vi "AuMT8852B Single Payload Frequency.vi"(5 "Frequency (2441 MHz)":dbl=2441.0, 7 "Set/Get (Set)":enum16{"Set", "Get"}(ring), 8 "error in (no error)":errorcluster, 9 "Type (TX)":enum16{"TX", "RX"}(ring), 10 "Script (3)":i32=3, 11 "VISA session":refnum<visa-resource-name>) -> (0 "error out":errorcluster, 2 "error code":i32, 3 "VISA session out":refnum<visa-resource-name>, 4 "Frequency out":dbl=2441.0)   [LabVIEW 2017]
doc: "Anritsu MT8850 Bluetooth Tester\n\nDetermines the TX or RX frequency for Bluetooth tests (Carrier, Sensitivity, etc.) whose scripts are set to Single Payload mode.\n\nINPUTS\n Set/Get - whether the value is being sent to or retrieved from the instrument.\n Script - the script to access.\n Type - whether the specified frequency is the TX or RX frequency.\n Frequency - value to be used in Single Payload mode.\n\nOUTPUTS\n Frequency out - value currently being used in Single Payload mode."
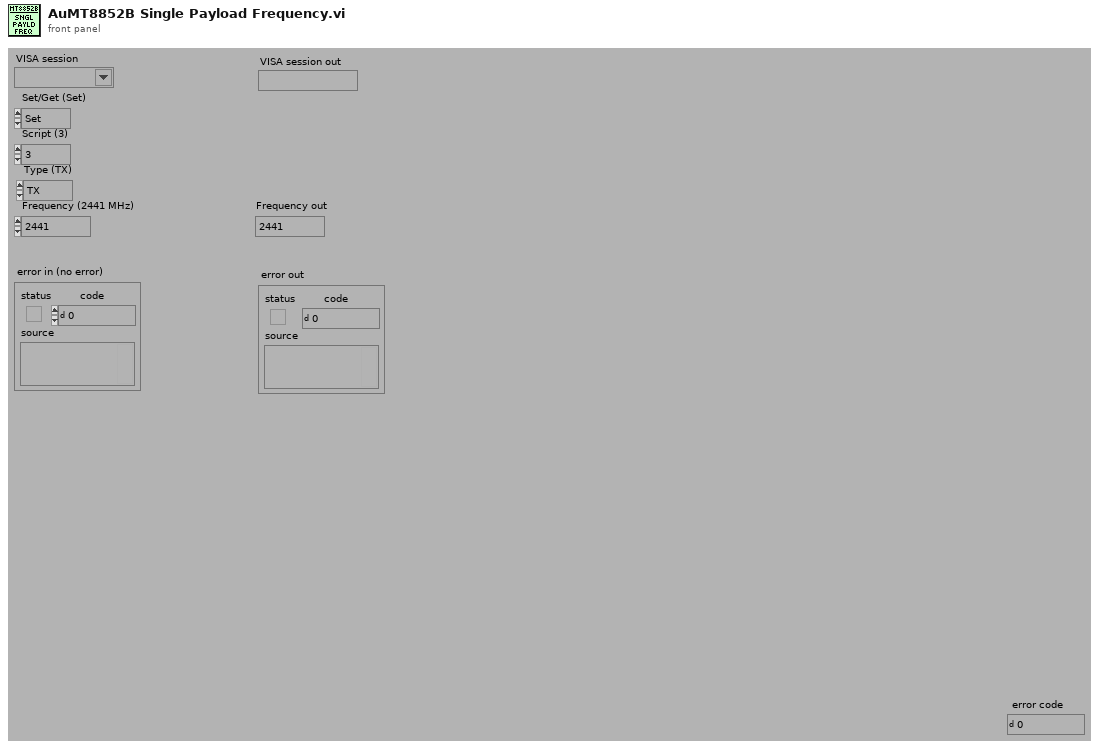
[diagram p1: front panel]
types:
  T1 = enum16{"Simulate", "Range check", "Cache", "Query instrument status"}
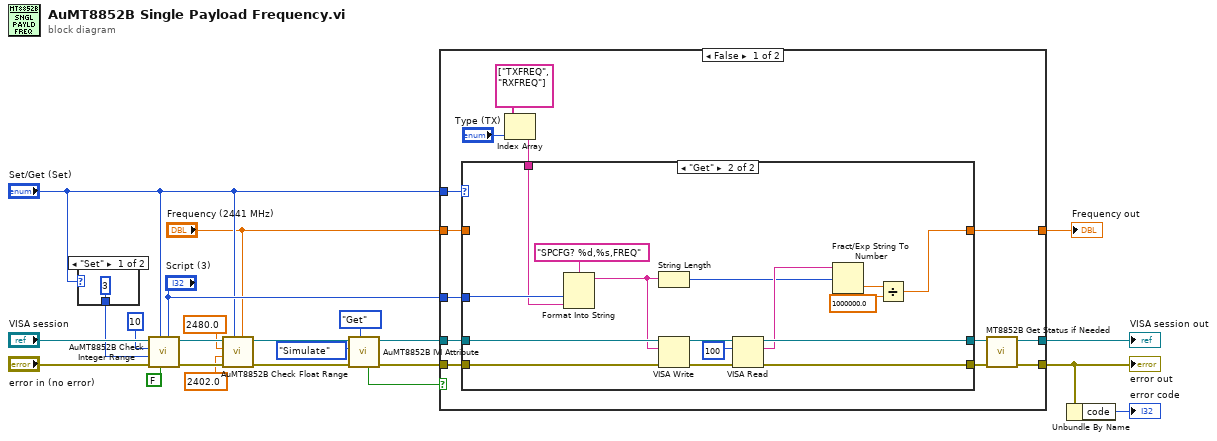
[diagram p0: block diagram]
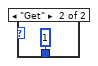
[diagram p2: hidden frame]
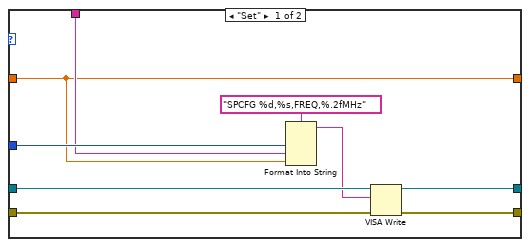
[diagram p3: hidden frame]
diagram:
  n1 = case shown="\"Set\"" "Set/Get (Set)" {
    tunnel: [3 1] -> w19
    frame "Set" {
    }
    frame "Get" {
    }
  }
  n2 = call <instrlib>:"AuMT8852B Check Integer Range.vi"("Value (0)"="Script (3)", "Check IVI flag first? (T)"=FALSE, "Set/Get (Set)"="Set/Get (Set)", "error in (no error)"="error in (no error)", "Lower limit (-1)"=w19, "Upper limit (1)"=10, "VISA session"="VISA session") -> ("error out"=w8:errorcluster, "VISA session out"=w7:refnum<visa-resource-name>)  [unwired: 3 in]
  n3 = call <instrlib>:"AuMT8852B Check Float Range.vi"("Value (0)"="Frequency (2441 MHz)", "Set/Get (Set)"="Set/Get (Set)", "error in (no error)"=w8, "Lower limit (-1)"=2402.0, "Upper limit (1)"=2480.0, "VISA session"=w7) -> ("error out"=w6:errorcluster, "VISA session out"=w5:refnum<visa-resource-name>)  [unwired: 4 in]
  n4 = call <instrlib>:"AuMT8852B IVI Attribute.vi"("Set/Get (Set)"=enum16{"Set", "Get"}."Get", "error in (no error)"=w6, "Flag (Simulate)"=T1."Simulate", "VISA session"=w5) -> ("error out"=w17:errorcluster, "VISA session out"=w18:refnum<visa-resource-name>, "Value out"=w14:bool)  [unwired: 5 in]
  n5 = case shown="False" w14 {
    tunnel: "Set/Get (Set)" -> [w38 _]
    tunnel: [w32 w65] -> w11
    tunnel: [w33 w66] -> w23
    tunnel: w18 -> [w37 w66]
    tunnel: w17 -> [w36 w65]
    tunnel: "Script (3)" -> [w31 _]
    tunnel: "Frequency (2441 MHz)" -> [w30 w64]
    tunnel: [w29 w64] -> w9
    frame False {
      n6 = Index Array(array=string[] ["TXFREQ", "RXFREQ"] ("Array Constant"), index="Type (TX)") -> (element=w26:string)
      n7 = case shown="\"Get\"" w38 {
        tunnel: [w44 w57] -> w34
        tunnel: [w45 w58] -> w35
        tunnel: w37 -> [w47 w63]
        tunnel: w36 -> [w46 w62]
        tunnel: w31 -> [w41 w55]
        tunnel: w30 -> [w39 _]
        tunnel: [w39 w48] -> w29
        tunnel: w26 -> [w40 w53]
        frame "Set" {
          n8 = Format Into String(format string="SPCFG %d,%s,FREQ,%.2fMHz" ("Format String"), w41, w40, w39) -> (resulting string=w42:string)  [unwired: 2 in, 1 out]
          n9 = VISA Write(VISA resource name=w47, write buffer=w42, error in (no error)=w46) -> (VISA resource name out=w45:refnum<visa-resource-name>, error out=w44:errorcluster)  [unwired: 1 out]
        }
        frame "Get" {
          n10 = Format Into String(format string="SPCFG? %d,%s,FREQ" ("Format String"), w55, w53) -> (resulting string=w54:string)  [unwired: 2 in, 1 out]
          n11 = String Length(string=w54) -> (length=w51:i32)
          n12 = VISA Write(VISA resource name=w63, write buffer=w54, error in (no error)=w62) -> (VISA resource name out=w61:refnum<visa-resource-name>, error out=w59:errorcluster)  [unwired: 1 out]
          n13 = VISA Read(VISA resource name=w61, byte count=u32 100 ("byte count (0)"), error in (no error)=w59) -> (VISA resource name out=w58:refnum<visa-resource-name>, read buffer=w52:string, error out=w57:errorcluster)  [unwired: 1 out]
          n14 = Fract/Exp String To Number(string=w52, offset=w51) -> (number=w50:dbl)  [unwired: 2 in, 1 out]
          n15 = Divide(x=w50, y=1000000.0) -> (x/y=w48:dbl)
        }
      }
      n16 = call <instrlib>:"MT8852B Get Status if Needed.vi"("error in (no error)"=w34, "VISA session"=w35) -> ("error out"=w32:errorcluster, "VISA session out"=w33:refnum<visa-resource-name>)  [unwired: 8 in]
    }
    frame True {
    }
  }
  "error out" <- w11
  "VISA session out" <- w23
  "Frequency out" <- w9
  n17 = Unbundle By Name(w11) -> ("code"=→"error code":i32)
